vi "DriverStationPushData.vi"   [LabVIEW 2019]
uses:
  1d2691cc-8b61-4dfb-bfb4-1b6bae38663e.vi
  d9edbeaf-af59-42c1-bcfe-b3e6a954c0a3.vi
  6bbe7408-9fb7-4578-b601-34b1cee8ce09.vi
  632ef858-b870-40c6-a12b-f40331275094.vi
  14719411-e5bb-4b11-9cb2-120e873c2e05.vi
  f1403ef2-33e1-4540-b343-9c65ccc4a920.vi
  7a513e6b-e498-46fb-8513-5316b3799954.vi
  69462ec0-83c8-47a3-81e1-900153dd9cc8.vi
  727b4c4a-f5c6-4f95-81f7-1339306d96f3.vi
  6d89053f-361e-40d0-a0fc-e8b482315cbe.vi
  fd2c5e75-7fca-48ad-946d-3f22856398bc.vi
  92d746a7-c9d7-4ce6-9695-b3a3d6975628.vi
  fd38028f-d706-4361-9c82-0aabc7820e26.vi
  3979fdd0-e033-4947-b603-c9c642562e84.vi
  226d75d0-f601-4189-bf0f-5b642a6ba181.vi
  e14e6ac2-87fa-4a9b-a8b4-52d3a40e65e0.vi
  d21848c3-9355-4e66-bfa9-f9c63735db0f.vi
  98ce0457-4a08-4b7b-804f-5414755b32f6.vi
  11425a44-503f-44e8-a25d-9300c812e48b.vi
  3419054f-dcb3-4bf8-a8cb-178e82c54ebb.vi
  b9084e3f-b8c4-4e28-9ab7-37ffbe7661f4.vi
  06b7b52c-29a6-4ba8-9c74-5b14680269ed.vi
  3f6f4240-928d-4554-8c23-d8546fc74eb4.vi
  2da9c99e-ca1f-4eea-96ff-37f6f5d11a4d.vi
  341659bb-139a-4f3b-a89e-b05073c7cc3d.vi
  3b85bbea-c33a-420d-8c98-77a31eb6e5f7.vi
  4d181bd6-f376-48f2-9f32-f633c6463892.vi
  3c552232-cdd6-41e6-be29-bb2e14258533.vi
  9a48e8f0-6742-4669-83f6-9efb9d3030e2.vi
  afaf0054-4057-4950-a884-559c498b9c60.vi
  3959e0c3-d817-4e3c-a233-589df82fb2a3.vi
  d45ba836-02d8-4962-bfcd-028c5a01eed1.vi
  8d6ec62f-e14d-40c9-b57a-da8c82ab6d12.vi
  578b3660-262a-43c4-999c-65651bac655b.vi
  constants.vi
  autoinfo.vi
  dsdata.vi
  <vilib>/Rock Robotics/Network Tables/NT Write String Array.vi
  sensors.vi
  <vilib>/Rock Robotics/Network Tables/NT Write Number.vi
  outputs.vi
  <vilib>/Rock Robotics/Network Tables/NT Write Boolean Array.vi
  <vilib>/Rock Robotics/Network Tables/NT Write Boolean.vi
  <vilib>/Rock Robotics/Network Tables/NT Write String.vi
  refnums.vi
  <vilib>/Rock Robotics/WPI/Utilities/WPI_GetSetVariantRefNum.vi
types:
  T1 = typedef "WPI_DriverStationRobotMode2.ctl" = enum16{"Autonomous Disabled", "Autonomous Enabled", "Teleop Disabled", "Teleop Enabled", "Disconnected", "Finish", "Test Disabled", "Test Enabled", "Emergency Stopped"}
  T2 = typedef "WPI_JoystickDevRef.ctl" = cluster{"Device":T3}
  T3 = typedef "WPI_JoystickDeviceEnum.ctl" = enum16{"USB 0", "USB 1", "USB 2", "USB 3", "USB 4", "USB 5"}
  T4 = typedef "WPI_DriverStationAllianceInfo.ctl" = enum16{"Red", "Blue", "Invalid"}
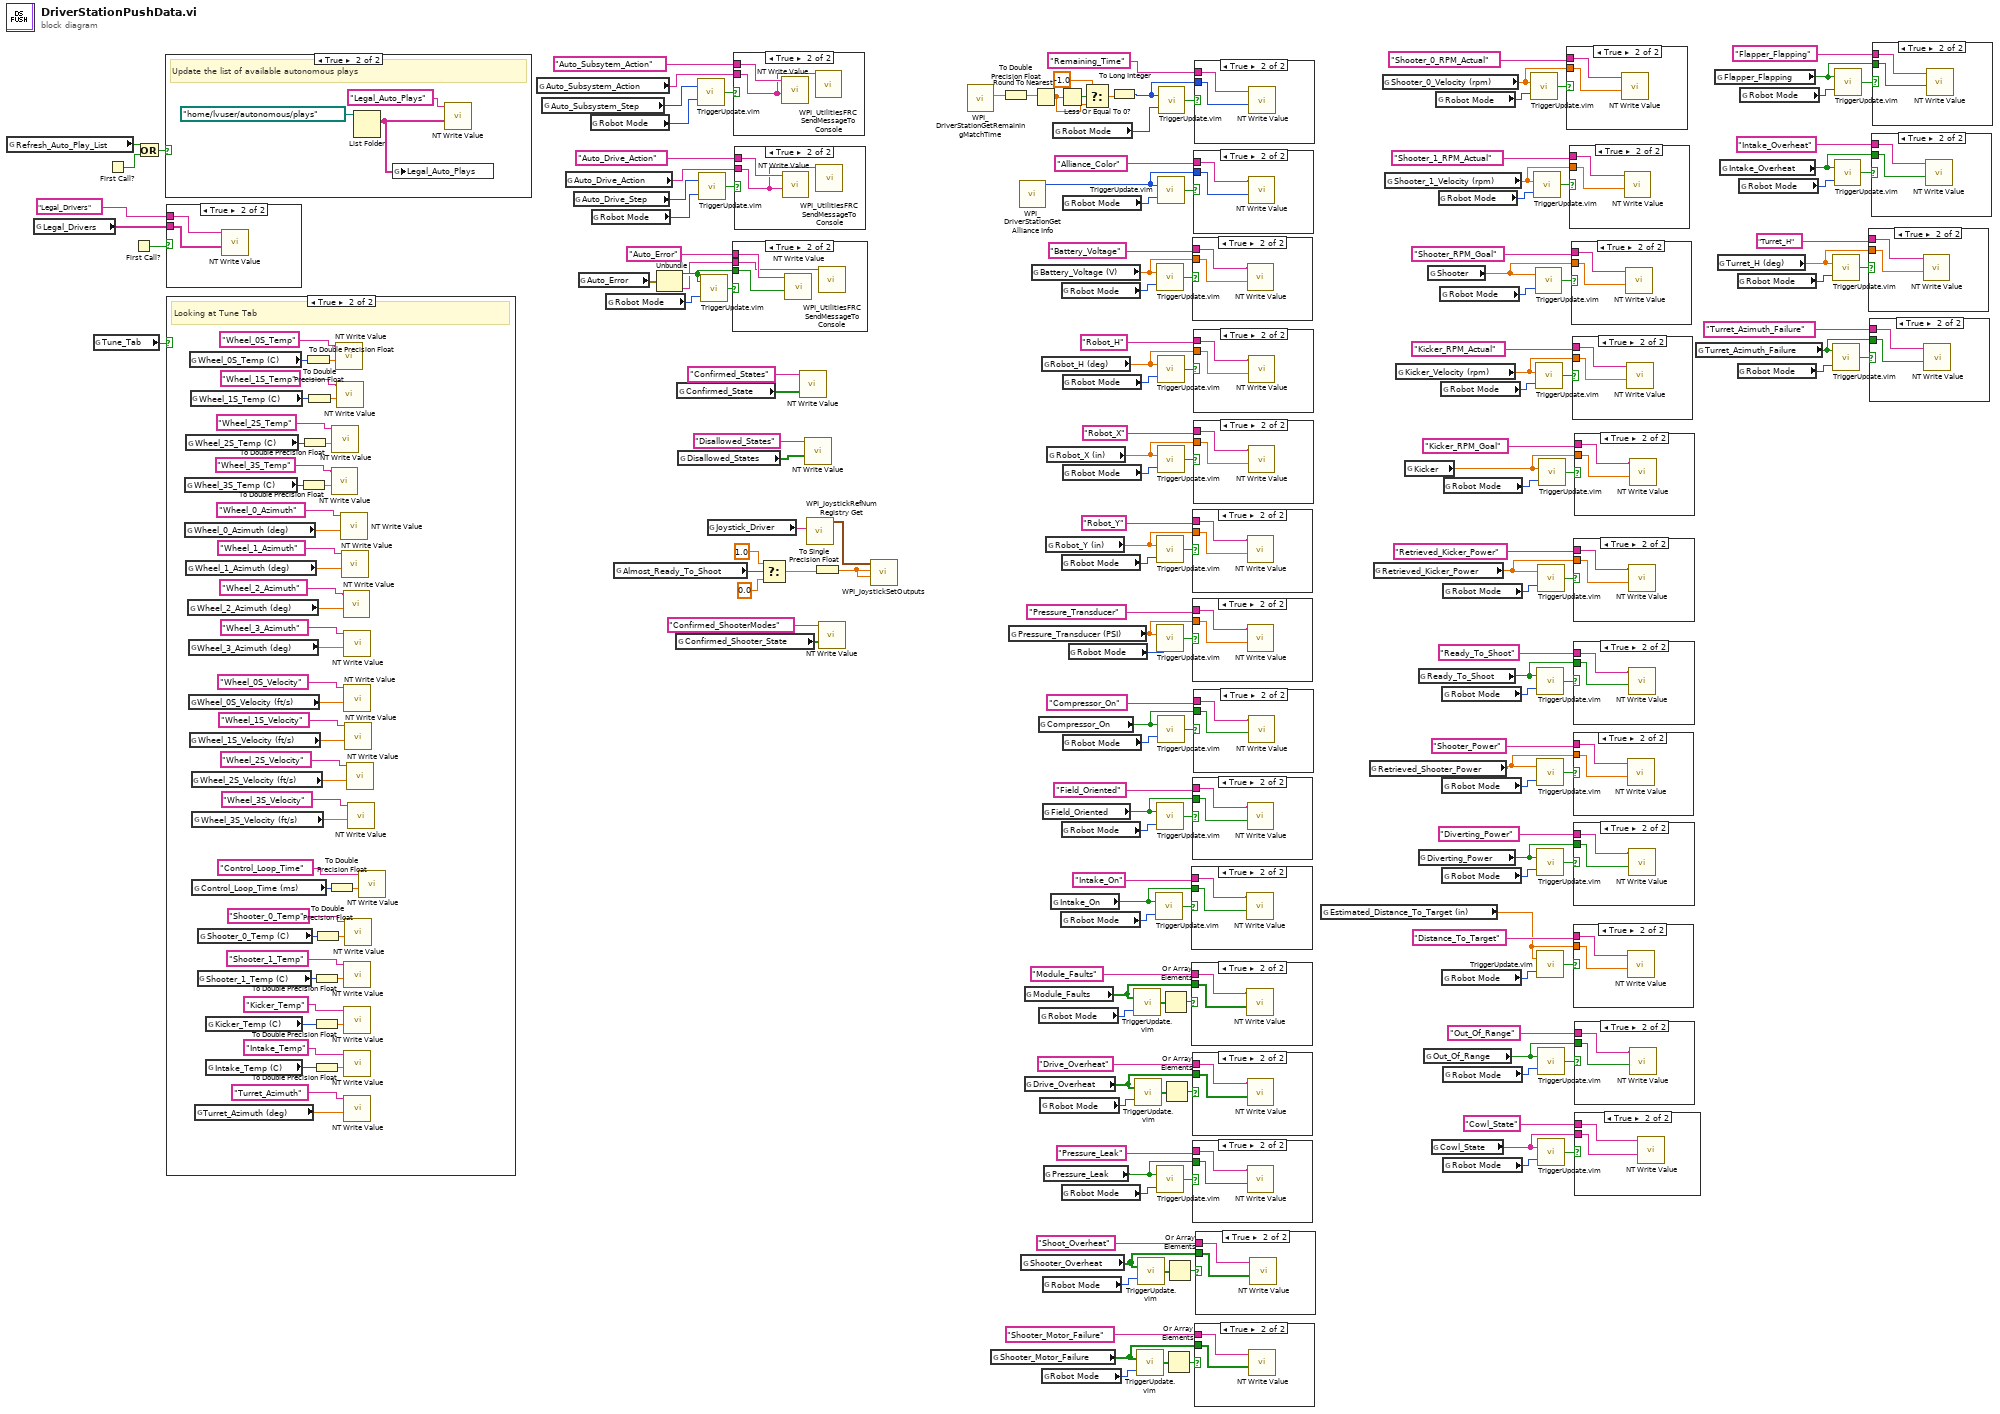
[diagram p0: block diagram]
diagram:
  n1 = global read "dsdata.vi" "Refresh_Auto_Play_List"() -> (w162:bool)
  n2 = global read "constants.vi" "Legal_Drivers"() -> (w159:string[])
  n3 = global read "dsdata.vi" "Tune_Tab"() -> (w142:bool)
  n4 = First Call?() -> (First Call?: T/F=w161:bool)
  n5 = First Call?() -> (First Call?: T/F=w157:bool)
  n6 = Or(x=w162, y=w161) -> (x .or. y?=w160:bool)
  n7 = case shown="True" w160 {
    frame False {
    }
    frame True {
      # "Update the list of available autonomous plays"
      n8 = List Folder(path=path "/home/lvuser/autonomous/plays") -> (filenames=w171:string[])  [unwired: 3 in, 3 out]
      n9 = global write "constants.vi" "Legal_Auto_Plays"(w171) -> ()
      n10 = call-poly <vilib>:"NT Write Value.vi"("String Array"=w171, "Name"="Legal_Auto_Plays") -> ()  [unwired: 9 in, 1 out]
    }
  }
  n11 = case shown="True" w157 {
    tunnel: w159 -> [_ w175]
    tunnel: "Legal_Drivers" ("Name") -> [_ w174]
    frame False {
    }
    frame True {
      n12 = call-poly <vilib>:"NT Write Value.vi"("String Array"=w175, "Name"=w174) -> ()  [unwired: 9 in, 1 out]
    }
  }
  n13 = case shown="True" w142 {
    frame False {
      # "Not Looking at Tune Tab"
    }
    frame True {
      # "Looking at Tune Tab"
      n14 = global read "sensors.vi" "Wheel_3S_Temp (C)"() -> (w200:u8)
      n15 = global read "sensors.vi" "Wheel_0_Azimuth (deg)"() -> (w217:dbl)
      n16 = global read "sensors.vi" "Wheel_2S_Temp (C)"() -> (w203:u8)
      n17 = global read "sensors.vi" "Wheel_1_Azimuth (deg)"() -> (w215:dbl)
      n18 = global read "sensors.vi" "Wheel_2_Azimuth (deg)"() -> (w213:dbl)
      n19 = global read "sensors.vi" "Wheel_3_Azimuth (deg)"() -> (w211:dbl)
      n20 = global read "sensors.vi" "Wheel_0S_Velocity (ft/s)"() -> (w191:dbl)
      n21 = global read "sensors.vi" "Wheel_0S_Temp (C)"() -> (w220:u8)
      n22 = global read "sensors.vi" "Wheel_1S_Velocity (ft/s)"() -> (w189:dbl)
      n23 = global read "sensors.vi" "Wheel_1S_Temp (C)"() -> (w206:u8)
      n24 = global read "sensors.vi" "Wheel_2S_Velocity (ft/s)"() -> (w187:dbl)
      n25 = global read "sensors.vi" "Wheel_3S_Velocity (ft/s)"() -> (w185:dbl)
      n26 = global read "sensors.vi" "Control_Loop_Time (ms)"() -> (w209:u32)
      n27 = global read "sensors.vi" "Turret_Azimuth (deg)"() -> (w177:dbl)
      n28 = global read "sensors.vi" "Shooter_1_Temp (C)"() -> (w194:u8)
      n29 = global read "sensors.vi" "Shooter_0_Temp (C)"() -> (w197:u8)
      n30 = global read "sensors.vi" "Kicker_Temp (C)"() -> (w183:u8)
      n31 = global read "sensors.vi" "Intake_Temp (C)"() -> (w180:u8)
      n32 = To Double Precision Float(number=w200) -> (double precision float=w198:dbl)
      n33 = To Double Precision Float(number=w203) -> (double precision float=w201:dbl)
      n34 = To Double Precision Float(number=w220) -> (double precision float=w218:dbl)
      n35 = To Double Precision Float(number=w206) -> (double precision float=w204:dbl)
      n36 = To Double Precision Float(number=w194) -> (double precision float=w192:dbl)
      n37 = To Double Precision Float(number=w183) -> (double precision float=w182:dbl)
      n38 = To Double Precision Float(number=w180) -> (double precision float=w179:dbl)
      n39 = To Double Precision Float(number=w197) -> (double precision float=w195:dbl)
      n40 = To Double Precision Float(number=w209) -> (double precision float=w207:dbl)
      n41 = call-poly <vilib>:"NT Write Value.vi"("Numeric"=w198, "Name"="Wheel_3S_Temp") -> ()  [unwired: 9 in, 1 out]
      n42 = call-poly <vilib>:"NT Write Value.vi"("Numeric"=w201, "Name"="Wheel_2S_Temp") -> ()  [unwired: 9 in, 1 out]
      n43 = call-poly <vilib>:"NT Write Value.vi"("Numeric"=w218, "Name"="Wheel_0S_Temp") -> ()  [unwired: 9 in, 1 out]
      n44 = call-poly <vilib>:"NT Write Value.vi"("Numeric"=w204, "Name"="Wheel_1S_Temp") -> ()  [unwired: 9 in, 1 out]
      n45 = call-poly <vilib>:"NT Write Value.vi"("Numeric"=w217, "Name"="Wheel_0_Azimuth") -> ()  [unwired: 9 in, 1 out]
      n46 = call-poly <vilib>:"NT Write Value.vi"("Numeric"=w215, "Name"="Wheel_1_Azimuth") -> ()  [unwired: 9 in, 1 out]
      n47 = call-poly <vilib>:"NT Write Value.vi"("Numeric"=w213, "Name"="Wheel_2_Azimuth") -> ()  [unwired: 9 in, 1 out]
      n48 = call-poly <vilib>:"NT Write Value.vi"("Numeric"=w211, "Name"="Wheel_3_Azimuth") -> ()  [unwired: 9 in, 1 out]
      n49 = call-poly <vilib>:"NT Write Value.vi"("Numeric"=w191, "Name"="Wheel_0S_Velocity") -> ()  [unwired: 9 in, 1 out]
      n50 = call-poly <vilib>:"NT Write Value.vi"("Numeric"=w192, "Name"="Shooter_1_Temp") -> ()  [unwired: 9 in, 1 out]
      n51 = call-poly <vilib>:"NT Write Value.vi"("Numeric"=w182, "Name"="Kicker_Temp") -> ()  [unwired: 9 in, 1 out]
      n52 = call-poly <vilib>:"NT Write Value.vi"("Numeric"=w179, "Name"="Intake_Temp") -> ()  [unwired: 9 in, 1 out]
      n53 = call-poly <vilib>:"NT Write Value.vi"("Numeric"=w177, "Name"="Turret_Azimuth") -> ()  [unwired: 9 in, 1 out]
      n54 = call-poly <vilib>:"NT Write Value.vi"("Numeric"=w189, "Name"="Wheel_1S_Velocity") -> ()  [unwired: 9 in, 1 out]
      n55 = call-poly <vilib>:"NT Write Value.vi"("Numeric"=w195, "Name"="Shooter_0_Temp") -> ()  [unwired: 9 in, 1 out]
      n56 = call-poly <vilib>:"NT Write Value.vi"("Numeric"=w187, "Name"="Wheel_2S_Velocity") -> ()  [unwired: 9 in, 1 out]
      n57 = call-poly <vilib>:"NT Write Value.vi"("Numeric"=w185, "Name"="Wheel_3S_Velocity") -> ()  [unwired: 9 in, 1 out]
      n58 = call-poly <vilib>:"NT Write Value.vi"("Numeric"=w207, "Name"="Control_Loop_Time") -> ()  [unwired: 9 in, 1 out]
    }
  }
  n59 = global read "autoinfo.vi" "Auto_Subsystem_Action"() -> (w164:string)
  n60 = global read "autoinfo.vi" "Auto_Subsystem_Step"() -> (w85:i32)
  n61 = global read "autoinfo.vi" "Auto_Drive_Action"() -> (w168:string)
  n62 = global read "autoinfo.vi" "Auto_Drive_Step"() -> (w84:i32)
  n63 = global read "autoinfo.vi" "Auto_Error"() -> (w92:errorcluster)
  n64 = global read "dsdata.vi" "Robot Mode"() -> (w166:T1)
  n65 = global read "dsdata.vi" "Robot Mode"() -> (w170:T1)
  n66 = global read "dsdata.vi" "Robot Mode"() -> (w95:T1)
  n67 = global read "outputs.vi" "Almost_Ready_To_Shoot"() -> (w73:bool)
  n68 = Unbundle(w92) -> ("status"=w91:bool, "source"=w90:string)  [unwired: 1 out]
  n69 = global read "outputs.vi" "Confirmed_Shooter_State"() -> (w50:bool[])
  n70 = global read "outputs.vi" "Confirmed_State"() -> (w128:bool[])
  n71 = global read "constants.vi" "Disallowed_States"() -> (w126:bool[])
  n72 = call "TriggerUpdate.vim"("Robot Mode"=w166, "Trigger"=w85) -> ("Update"=w165:bool)
  n73 = call "TriggerUpdate.vim"("Robot Mode"=w170, "Trigger"=w84) -> ("Update"=w169:bool)
  n74 = call "TriggerUpdate.vim"("Robot Mode"=w95, "Trigger"=w91) -> ("Update"=w94:bool)
  n75 = global read "refnums.vi" "Joystick_Driver"() -> (w79:string)
  n76 = case shown="True" w94 {
    tunnel: w91 -> [_ w222]
    tunnel: "Auto_Error" ("Name") -> [_ w223]
    tunnel: w90 -> [_ w221]
    frame False {
    }
    frame True {
      n77 = call-poly <vilib>:"NT Write Value.vi"("Boolean"=w222, "Name"=w223) -> ()  [unwired: 9 in, 1 out]
      n78 = call <vilib>:"WPI_UtilitiesFRC SendMessageToConsole.vi"("Message"=w221) -> ()  [unwired: 14 in, 1 out]
    }
  }
  n79 = case shown="True" w165 {
    tunnel: w164 -> [_ w224]
    tunnel: "Auto_Subsytem_Action" ("Name") -> [_ w225]
    frame False {
    }
    frame True {
      n80 = call-poly <vilib>:"NT Write Value.vi"("String"=w224, "Name"=w225) -> ()  [unwired: 9 in, 1 out]
      n81 = call <vilib>:"WPI_UtilitiesFRC SendMessageToConsole.vi"("Message"=w224) -> ()  [unwired: 14 in, 1 out]
    }
  }
  n82 = case shown="True" w169 {
    tunnel: w168 -> [_ w226]
    tunnel: "Auto_Drive_Action" ("Name") -> [_ w227]
    frame False {
    }
    frame True {
      n83 = call-poly <vilib>:"NT Write Value.vi"("String"=w226, "Name"=w227) -> ()  [unwired: 9 in, 1 out]
      n84 = call <vilib>:"WPI_UtilitiesFRC SendMessageToConsole.vi"("Message"=w226) -> ()  [unwired: 14 in, 1 out]
    }
  }
  n85 = Select(t=1.0, s=w73, f=0.0) -> (s? t:f=w81:dbl)
  n86 = call-poly <vilib>:"NT Write Value.vi"("Boolean Array"=w128, "Name"="Confirmed_States") -> ()  [unwired: 9 in, 1 out]
  n87 = call-poly <vilib>:"NT Write Value.vi"("Boolean Array"=w126, "Name"="Disallowed_States") -> ()  [unwired: 9 in, 1 out]
  n88 = call <vilib>:"WPI_JoystickRefNum Registry Get.vi"("refnum name"=w79) -> ("JoystickDevRef"=w78:T2)  [unwired: 9 in, 1 out]
  n89 = To Single Precision Float(number=w81) -> (single precision float=w80:sgl)
  n90 = call-poly <vilib>:"NT Write Value.vi"("Boolean Array"=w50, "Name"="Confirmed_ShooterModes") -> ()  [unwired: 9 in, 1 out]
  n91 = call <vilib>:"WPI_JoystickSetOutputs.vi"("Right Rumble"=w80, "Left Rumble"=w80, "JoystickDevRef"=w78) -> ()  [unwired: 7 in, 2 out]
  n92 = call <vilib>:"WPI_DriverStationGetRemainingMatchTime.vi"() -> ("Match Time(s)"=w151:sgl)  [unwired: 10 in, 1 out]
  n93 = global read "sensors.vi" "Shooter_Motor_Failure"() -> (w43:bool[])
  n94 = To Double Precision Float(number=w151) -> (double precision float=w156:dbl)
  n95 = global read "sensors.vi" "Pressure_Transducer (PSI)"() -> (w122:dbl)
  n96 = call <vilib>:"WPI_DriverStationGet Alliance Info.vi"() -> ("Alliance"=w114:T4)  [unwired: 6 in, 5 out]
  n97 = global read "sensors.vi" "Shooter_Overheat"() -> (w62:bool[])
  n98 = global read "sensors.vi" "Module_Faults"() -> (w107:bool[])
  n99 = global read "sensors.vi" "Drive_Overheat"() -> (w102:bool[])
  n100 = global read "sensors.vi" "Battery_Voltage (V)"() -> (w147:dbl)
  n101 = Round To Nearest(number=w156) -> (nearest integer value=w154:dbl)
  n102 = global read "sensors.vi" "Compressor_On"() -> (w118:bool)
  n103 = global read "dsdata.vi" "Robot Mode"() -> (w109:T1)
  n104 = global read "dsdata.vi" "Robot Mode"() -> (w104:T1)
  n105 = global read "sensors.vi" "Robot_H (deg)"() -> (w138:dbl)
  n106 = global read "dsdata.vi" "Robot Mode"() -> (w45:T1)
  n107 = global read "outputs.vi" "Field_Oriented"() -> (w110:bool)
  n108 = global read "dsdata.vi" "Robot Mode"() -> (w64:T1)
  n109 = global read "sensors.vi" "Pressure_Leak"() -> (w96:bool)
  n110 = global read "sensors.vi" "Robot_Y (in)"() -> (w130:dbl)
  n111 = global read "sensors.vi" "Robot_X (in)"() -> (w134:dbl)
  n112 = global read "outputs.vi" "Intake_On"() -> (w86:bool)
  n113 = global read "dsdata.vi" "Robot Mode"() -> (w145:T1)
  n114 = Less Or Equal To 0?(x=w154) -> (x <= 0?=w155:bool)
  n115 = global read "dsdata.vi" "Robot Mode"() -> (w88:T1)
  n116 = global read "dsdata.vi" "Robot Mode"() -> (w149:T1)
  n117 = global read "dsdata.vi" "Robot Mode"() -> (w132:T1)
  n118 = global read "dsdata.vi" "Robot Mode"() -> (w112:T1)
  n119 = global read "dsdata.vi" "Robot Mode"() -> (w98:T1)
  n120 = global read "dsdata.vi" "Robot Mode"() -> (w116:T1)
  n121 = global read "dsdata.vi" "Robot Mode"() -> (w140:T1)
  n122 = global read "dsdata.vi" "Robot Mode"() -> (w136:T1)
  n123 = global read "dsdata.vi" "Robot Mode"() -> (w120:T1)
  n124 = global read "dsdata.vi" "Robot Mode"() -> (w124:T1)
  n125 = Select(t=-1.0, s=w155, f=w154) -> (s? t:f=w153:dbl)
  n126 = To Long Integer(number=w153) -> (32bit integer=w144:i32)
  n127 = call "TriggerUpdate.vim"("Robot Mode"=w109, "Trigger"=w107) -> ("Update"=w106:bool[])
  n128 = call "TriggerUpdate.vim"("Robot Mode"=w104, "Trigger"=w102) -> ("Update"=w101:bool[])
  n129 = call "TriggerUpdate.vim"("Robot Mode"=w45, "Trigger"=w43) -> ("Update"=w42:bool[])
  n130 = call "TriggerUpdate.vim"("Robot Mode"=w64, "Trigger"=w62) -> ("Update"=w61:bool[])
  n131 = call "TriggerUpdate.vim"("Robot Mode"=w88, "Trigger"=w86) -> ("Update"=w89:bool)
  n132 = call "TriggerUpdate.vim"("Robot Mode"=w149, "Trigger"=w147) -> ("Update"=w150:bool)
  n133 = call "TriggerUpdate.vim"("Robot Mode"=w132, "Trigger"=w130) -> ("Update"=w133:bool)
  n134 = call "TriggerUpdate.vim"("Robot Mode"=w124, "Trigger"=w122) -> ("Update"=w125:bool)
  n135 = call "TriggerUpdate.vim"("Robot Mode"=w112, "Trigger"=w110) -> ("Update"=w113:bool)
  n136 = call "TriggerUpdate.vim"("Robot Mode"=w98, "Trigger"=w96) -> ("Update"=w99:bool)
  n137 = call "TriggerUpdate.vim"("Robot Mode"=w116, "Trigger"=w114) -> ("Update"=w117:bool)
  n138 = call "TriggerUpdate.vim"("Robot Mode"=w140, "Trigger"=w138) -> ("Update"=w141:bool)
  n139 = call "TriggerUpdate.vim"("Robot Mode"=w136, "Trigger"=w134) -> ("Update"=w137:bool)
  n140 = call "TriggerUpdate.vim"("Robot Mode"=w120, "Trigger"=w118) -> ("Update"=w121:bool)
  n141 = call "TriggerUpdate.vim"("Robot Mode"=w145, "Trigger"=w144) -> ("Update"=w146:bool)
  n142 = Or Array Elements(Boolean array=w106) -> (logical OR=w105:bool)
  n143 = Or Array Elements(Boolean array=w101) -> (logical OR=w100:bool)
  n144 = Or Array Elements(Boolean array=w42) -> (logical OR=w41:bool)
  n145 = Or Array Elements(Boolean array=w61) -> (logical OR=w60:bool)
  n146 = case shown="True" w89 {
    tunnel: w86 -> [_ w229]
    tunnel: "Intake_On" ("Name") -> [_ w228]
    frame False {
    }
    frame True {
      n147 = call-poly <vilib>:"NT Write Value.vi"("Boolean"=w229, "Name"=w228) -> ()  [unwired: 9 in, 1 out]
    }
  }
  n148 = case shown="True" w105 {
    tunnel: w107 -> [_ w231]
    tunnel: "Module_Faults" ("Name") -> [_ w230]
    frame False {
    }
    frame True {
      n149 = call-poly <vilib>:"NT Write Value.vi"("Boolean Array"=w231, "Name"=w230) -> ()  [unwired: 9 in, 1 out]
    }
  }
  n150 = case shown="True" w150 {
    tunnel: w147 -> [_ w233]
    tunnel: "Battery_Voltage" ("Name") -> [_ w232]
    frame False {
    }
    frame True {
      n151 = call-poly <vilib>:"NT Write Value.vi"("Numeric"=w233, "Name"=w232) -> ()  [unwired: 9 in, 1 out]
    }
  }
  n152 = case shown="True" w133 {
    tunnel: w130 -> [_ w235]
    tunnel: "Robot_Y" ("Name") -> [_ w234]
    frame False {
    }
    frame True {
      n153 = call-poly <vilib>:"NT Write Value.vi"("Numeric"=w235, "Name"=w234) -> ()  [unwired: 9 in, 1 out]
    }
  }
  n154 = case shown="True" w125 {
    tunnel: w122 -> [_ w237]
    tunnel: "Pressure_Transducer" ("Name") -> [_ w236]
    frame False {
    }
    frame True {
      n155 = call-poly <vilib>:"NT Write Value.vi"("Numeric"=w237, "Name"=w236) -> ()  [unwired: 9 in, 1 out]
    }
  }
  n156 = case shown="True" w113 {
    tunnel: w110 -> [_ w239]
    tunnel: "Field_Oriented" ("Name") -> [_ w238]
    frame False {
    }
    frame True {
      n157 = call-poly <vilib>:"NT Write Value.vi"("Boolean"=w239, "Name"=w238) -> ()  [unwired: 9 in, 1 out]
    }
  }
  n158 = case shown="True" w100 {
    tunnel: w102 -> [_ w241]
    tunnel: "Drive_Overheat" ("Name") -> [_ w240]
    frame False {
    }
    frame True {
      n159 = call-poly <vilib>:"NT Write Value.vi"("Boolean Array"=w241, "Name"=w240) -> ()  [unwired: 9 in, 1 out]
    }
  }
  n160 = case shown="True" w99 {
    tunnel: w96 -> [_ w243]
    tunnel: "Pressure_Leak" ("Name") -> [_ w242]
    frame False {
    }
    frame True {
      n161 = call-poly <vilib>:"NT Write Value.vi"("Boolean"=w243, "Name"=w242) -> ()  [unwired: 9 in, 1 out]
    }
  }
  n162 = case shown="True" w117 {
    tunnel: w114 -> [_ w245]
    tunnel: "Alliance_Color" ("Name") -> [_ w244]
    frame False {
    }
    frame True {
      n163 = call-poly <vilib>:"NT Write Value.vi"("Numeric"=w245, "Name"=w244) -> ()  [unwired: 9 in, 1 out]
    }
  }
  n164 = case shown="True" w141 {
    tunnel: w138 -> [_ w247]
    tunnel: "Robot_H" ("Name") -> [_ w246]
    frame False {
    }
    frame True {
      n165 = call-poly <vilib>:"NT Write Value.vi"("Numeric"=w247, "Name"=w246) -> ()  [unwired: 9 in, 1 out]
    }
  }
  n166 = case shown="True" w137 {
    tunnel: w134 -> [_ w249]
    tunnel: "Robot_X" ("Name") -> [_ w248]
    frame False {
    }
    frame True {
      n167 = call-poly <vilib>:"NT Write Value.vi"("Numeric"=w249, "Name"=w248) -> ()  [unwired: 9 in, 1 out]
    }
  }
  n168 = case shown="True" w121 {
    tunnel: w118 -> [_ w251]
    tunnel: "Compressor_On" ("Name") -> [_ w250]
    frame False {
    }
    frame True {
      n169 = call-poly <vilib>:"NT Write Value.vi"("Boolean"=w251, "Name"=w250) -> ()  [unwired: 9 in, 1 out]
    }
  }
  n170 = case shown="True" w146 {
    tunnel: w144 -> [_ w253]
    tunnel: "Remaining_Time" ("Name") -> [_ w252]
    frame False {
    }
    frame True {
      n171 = call-poly <vilib>:"NT Write Value.vi"("Numeric"=w253, "Name"=w252) -> ()  [unwired: 9 in, 1 out]
    }
  }
  n172 = case shown="True" w41 {
    tunnel: w43 -> [_ w255]
    tunnel: "Shooter_Motor_Failure" ("Name") -> [_ w254]
    frame False {
    }
    frame True {
      n173 = call-poly <vilib>:"NT Write Value.vi"("Boolean Array"=w255, "Name"=w254) -> ()  [unwired: 9 in, 1 out]
    }
  }
  n174 = case shown="True" w60 {
    tunnel: w62 -> [_ w257]
    tunnel: "Shoot_Overheat" ("Name") -> [_ w256]
    frame False {
    }
    frame True {
      n175 = call-poly <vilib>:"NT Write Value.vi"("Boolean Array"=w257, "Name"=w256) -> ()  [unwired: 9 in, 1 out]
    }
  }
  n176 = global read "sensors.vi" "Estimated_Distance_To_Target (in)"() -> (w2:dbl)
  n177 = global read "sensors.vi" "Retrieved_Shooter_Power"() -> (w52:dbl)
  n178 = global read "outputs.vi" "Retrieved_Kicker_Power"() -> (w22:dbl)
  n179 = global read "sensors.vi" "Shooter_0_Velocity (rpm)"() -> (w74:dbl)
  n180 = global read "sensors.vi" "Shooter_1_Velocity (rpm)"() -> (w69:dbl)
  n181 = global read "sensors.vi" "Kicker_Velocity (rpm)"() -> (w26:dbl)
  n182 = global read "outputs.vi" "Kicker"() -> (w1:dbl)
  n183 = global read "outputs.vi" "Ready_To_Shoot"() -> (w56:bool)
  n184 = global read "outputs.vi" "Diverting_Power"() -> (w46:bool)
  n185 = global read "outputs.vi" "Out_Of_Range"() -> (w34:bool)
  n186 = global read "outputs.vi" "Shooter"() -> (w65:dbl)
  n187 = global read "outputs.vi" "Cowl_State"() -> (w30:string)
  n188 = global read "dsdata.vi" "Robot Mode"() -> (w76:T1)
  n189 = global read "dsdata.vi" "Robot Mode"() -> (w71:T1)
  n190 = global read "dsdata.vi" "Robot Mode"() -> (w67:T1)
  n191 = global read "dsdata.vi" "Robot Mode"() -> (w28:T1)
  n192 = global read "dsdata.vi" "Robot Mode"() -> (w58:T1)
  n193 = global read "dsdata.vi" "Robot Mode"() -> (w54:T1)
  n194 = global read "dsdata.vi" "Robot Mode"() -> (w48:T1)
  n195 = global read "dsdata.vi" "Robot Mode"() -> (w39:T1)
  n196 = global read "dsdata.vi" "Robot Mode"() -> (w24:T1)
  n197 = global read "dsdata.vi" "Robot Mode"() -> (w36:T1)
  n198 = global read "dsdata.vi" "Robot Mode"() -> (w32:T1)
  n199 = global read "dsdata.vi" "Robot Mode"() -> (w20:T1)
  n200 = call "TriggerUpdate.vim"("Robot Mode"=w76, "Trigger"=w74) -> ("Update"=w77:bool)
  n201 = call "TriggerUpdate.vim"("Robot Mode"=w71, "Trigger"=w69) -> ("Update"=w72:bool)
  n202 = call "TriggerUpdate.vim"("Robot Mode"=w67, "Trigger"=w65) -> ("Update"=w68:bool)
  n203 = call "TriggerUpdate.vim"("Robot Mode"=w28, "Trigger"=w26) -> ("Update"=w29:bool)
  n204 = call "TriggerUpdate.vim"("Robot Mode"=w58, "Trigger"=w56) -> ("Update"=w59:bool)
  n205 = call "TriggerUpdate.vim"("Robot Mode"=w54, "Trigger"=w52) -> ("Update"=w55:bool)
  n206 = call "TriggerUpdate.vim"("Robot Mode"=w48, "Trigger"=w46) -> ("Update"=w49:bool)
  n207 = call "TriggerUpdate.vim"("Robot Mode"=w39, "Trigger"=w2) -> ("Update"=w40:bool)
  n208 = call "TriggerUpdate.vim"("Robot Mode"=w24, "Trigger"=w22) -> ("Update"=w25:bool)
  n209 = call "TriggerUpdate.vim"("Robot Mode"=w36, "Trigger"=w34) -> ("Update"=w37:bool)
  n210 = call "TriggerUpdate.vim"("Robot Mode"=w32, "Trigger"=w30) -> ("Update"=w33:bool)
  n211 = call "TriggerUpdate.vim"("Robot Mode"=w20, "Trigger"=w1) -> ("Update"=w21:bool)
  n212 = case shown="True" w77 {
    tunnel: w74 -> [_ w259]
    tunnel: "Shooter_0_RPM_Actual" ("Name") -> [_ w258]
    frame False {
    }
    frame True {
      n213 = call-poly <vilib>:"NT Write Value.vi"("Numeric"=w259, "Name"=w258) -> ()  [unwired: 9 in, 1 out]
    }
  }
  n214 = case shown="True" w72 {
    tunnel: w69 -> [_ w261]
    tunnel: "Shooter_1_RPM_Actual" ("Name") -> [_ w260]
    frame False {
    }
    frame True {
      n215 = call-poly <vilib>:"NT Write Value.vi"("Numeric"=w261, "Name"=w260) -> ()  [unwired: 9 in, 1 out]
    }
  }
  n216 = case shown="True" w68 {
    tunnel: w65 -> [_ w263]
    tunnel: "Shooter_RPM_Goal" ("Name") -> [_ w262]
    frame False {
    }
    frame True {
      n217 = call-poly <vilib>:"NT Write Value.vi"("Numeric"=w263, "Name"=w262) -> ()  [unwired: 9 in, 1 out]
    }
  }
  n218 = case shown="True" w29 {
    tunnel: w26 -> [_ w265]
    tunnel: "Kicker_RPM_Actual" ("Name") -> [_ w264]
    frame False {
    }
    frame True {
      n219 = call-poly <vilib>:"NT Write Value.vi"("Numeric"=w265, "Name"=w264) -> ()  [unwired: 9 in, 1 out]
    }
  }
  n220 = case shown="True" w55 {
    tunnel: w52 -> [_ w267]
    tunnel: "Shooter_Power" ("Name") -> [_ w266]
    frame False {
    }
    frame True {
      n221 = call-poly <vilib>:"NT Write Value.vi"("Numeric"=w267, "Name"=w266) -> ()  [unwired: 9 in, 1 out]
    }
  }
  n222 = case shown="True" w40 {
    tunnel: w2 -> [_ w269]
    tunnel: "Distance_To_Target" ("Name") -> [_ w268]
    frame False {
    }
    frame True {
      n223 = call-poly <vilib>:"NT Write Value.vi"("Numeric"=w269, "Name"=w268) -> ()  [unwired: 9 in, 1 out]
    }
  }
  n224 = case shown="True" w25 {
    tunnel: w22 -> [_ w271]
    tunnel: "Retrieved_Kicker_Power" ("Name") -> [_ w270]
    frame False {
    }
    frame True {
      n225 = call-poly <vilib>:"NT Write Value.vi"("Numeric"=w271, "Name"=w270) -> ()  [unwired: 9 in, 1 out]
    }
  }
  n226 = case shown="True" w59 {
    tunnel: w56 -> [_ w273]
    tunnel: "Ready_To_Shoot" ("Name") -> [_ w272]
    frame False {
    }
    frame True {
      n227 = call-poly <vilib>:"NT Write Value.vi"("Boolean"=w273, "Name"=w272) -> ()  [unwired: 9 in, 1 out]
    }
  }
  n228 = case shown="True" w49 {
    tunnel: w46 -> [_ w275]
    tunnel: "Diverting_Power" ("Name") -> [_ w274]
    frame False {
    }
    frame True {
      n229 = call-poly <vilib>:"NT Write Value.vi"("Boolean"=w275, "Name"=w274) -> ()  [unwired: 9 in, 1 out]
    }
  }
  n230 = case shown="True" w21 {
    tunnel: w1 -> [_ w277]
    tunnel: "Kicker_RPM_Goal" ("Name") -> [_ w276]
    frame False {
    }
    frame True {
      n231 = call-poly <vilib>:"NT Write Value.vi"("Numeric"=w277, "Name"=w276) -> ()  [unwired: 9 in, 1 out]
    }
  }
  n232 = case shown="True" w37 {
    tunnel: w34 -> [_ w279]
    tunnel: "Out_Of_Range" ("Name") -> [_ w278]
    frame False {
    }
    frame True {
      n233 = call-poly <vilib>:"NT Write Value.vi"("Boolean"=w279, "Name"=w278) -> ()  [unwired: 9 in, 1 out]
    }
  }
  n234 = case shown="True" w33 {
    tunnel: w30 -> [_ w280]
    tunnel: "Cowl_State" ("Name") -> [_ w281]
    frame False {
    }
    frame True {
      n235 = call-poly <vilib>:"NT Write Value.vi"("String"=w280, "Name"=w281) -> ()  [unwired: 9 in, 1 out]
    }
  }
  n236 = global read "sensors.vi" "Turret_Azimuth_Failure"() -> (w3:bool)
  n237 = global read "outputs.vi" "Flapper_Flapping"() -> (w15:bool)
  n238 = global read "sensors.vi" "Turret_H (deg)"() -> (w7:dbl)
  n239 = global read "sensors.vi" "Intake_Overheat"() -> (w11:bool)
  n240 = global read "dsdata.vi" "Robot Mode"() -> (w9:T1)
  n241 = global read "dsdata.vi" "Robot Mode"() -> (w5:T1)
  n242 = global read "dsdata.vi" "Robot Mode"() -> (w13:T1)
  n243 = global read "dsdata.vi" "Robot Mode"() -> (w17:T1)
  n244 = call "TriggerUpdate.vim"("Robot Mode"=w9, "Trigger"=w7) -> ("Update"=w10:bool)
  n245 = call "TriggerUpdate.vim"("Robot Mode"=w5, "Trigger"=w3) -> ("Update"=w6:bool)
  n246 = call "TriggerUpdate.vim"("Robot Mode"=w13, "Trigger"=w11) -> ("Update"=w14:bool)
  n247 = call "TriggerUpdate.vim"("Robot Mode"=w17, "Trigger"=w15) -> ("Update"=w18:bool)
  n248 = case shown="True" w10 {
    tunnel: w7 -> [_ w283]
    tunnel: "Turret_H" ("Name") -> [_ w282]
    frame False {
    }
    frame True {
      n249 = call-poly <vilib>:"NT Write Value.vi"("Numeric"=w283, "Name"=w282) -> ()  [unwired: 9 in, 1 out]
    }
  }
  n250 = case shown="True" w6 {
    tunnel: w3 -> [_ w285]
    tunnel: "Turret_Azimuth_Failure" ("Name") -> [_ w284]
    frame False {
    }
    frame True {
      n251 = call-poly <vilib>:"NT Write Value.vi"("Boolean"=w285, "Name"=w284) -> ()  [unwired: 9 in, 1 out]
    }
  }
  n252 = case shown="True" w14 {
    tunnel: w11 -> [_ w287]
    tunnel: "Intake_Overheat" ("Name") -> [_ w286]
    frame False {
    }
    frame True {
      n253 = call-poly <vilib>:"NT Write Value.vi"("Boolean"=w287, "Name"=w286) -> ()  [unwired: 9 in, 1 out]
    }
  }
  n254 = case shown="True" w18 {
    tunnel: w15 -> [_ w289]
    tunnel: "Flapper_Flapping" ("Name") -> [_ w288]
    frame False {
    }
    frame True {
      n255 = call-poly <vilib>:"NT Write Value.vi"("Boolean"=w289, "Name"=w288) -> ()  [unwired: 9 in, 1 out]
    }
  }
